vi "HasNext.vi"(8 "error in (no error)":errorcluster, 11 "CompositeIterator":refnum<class "CompositeIterator.lvclass">) -> (0 "error out":errorcluster, 2 "HasNext?(False)":bool, 3 "CompositeIterator Out":refnum<class "CompositeIterator.lvclass">)   [LabVIEW 2015, in "CompositeIterator.lvclass"]
uses:
  CompositeIterator.lvclass
  Interface/Iterator.lvclass
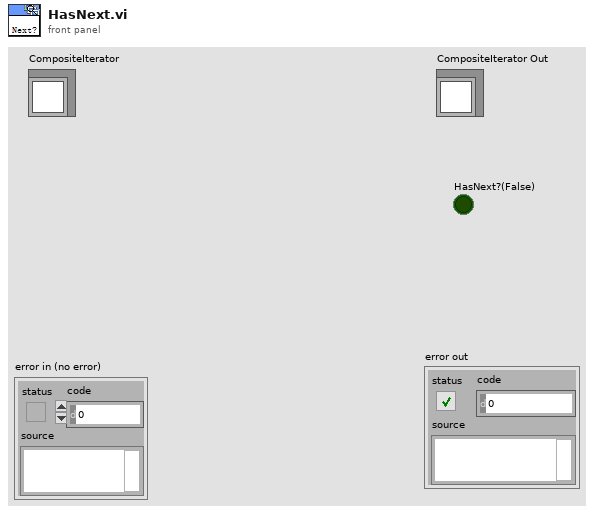
[diagram p1: front panel]
types:
  T1 = typedef "CompositeIterator.lvclass/ObjectAttributes.ctl" = cluster{"Stack":refnum<queue>}
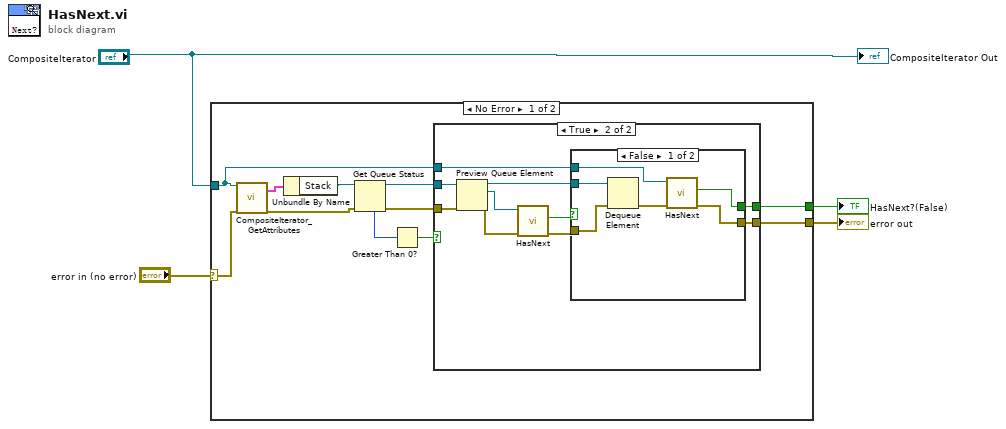
[diagram p0: block diagram]
diagram:
  n1 = case shown="No Error" "error in (no error)" {
    selector: "error in (no error)" -> [w7 w36]
    tunnel: "CompositeIterator" -> [w8 _]
    tunnel: [w11 _] -> w4
    tunnel: [w10 w36] -> w3
    frame No Error {
      n2 = call "CompositeIterator_GetAttributes.vi"("reference in"=w8, "error in (no error)"=w7) -> ("Data"=w6:T1, "error out"=w5:errorcluster)  [unwired: 14 in, 2 out]
      n3 = Unbundle By Name(w6) -> ("Stack"=w9:refnum<queue>)
      n4 = Get Queue Status(queue=w9, error in (no error)=w5) -> (queue out=w12:refnum<queue>, error out=w13:errorcluster, # elements in queue=w15:i32)  [unwired: 1 in, 5 out]
      n5 = Greater Than 0?(x=w15) -> (x > 0?=w14:bool)
      n6 = case shown="True" w14 {
        selector: w14 -> [w17 _]
        tunnel: w13 -> [w16 w26]
        tunnel: w12 -> [_ w27]
        tunnel: [w17 w24] -> w11
        tunnel: [w16 w23] -> w10
        tunnel: w8 -> [_ w22]
        frame False {
        }
        frame True {
          n7 = Preview Queue Element(queue=w27, error in (no error)=w26) -> (queue out=w25:refnum<queue>, element=w21:refnum<class "Iterator.lvclass">, error out=w20:errorcluster)  [unwired: 1 in, 1 out]
          n8 = call-dynamic "HasNext.vi"("error in (no error)"=w20, "Iterator"=w21) -> ("error out"=w18:errorcluster, "HasNext?(False)"=w19:bool)  [unwired: 7 in, 1 out]
          n9 = case shown="False" w19 {
            selector: w19 -> [_ w34]
            tunnel: w18 -> [w33 w35]
            tunnel: w25 -> [w32 _]
            tunnel: [w28 w34] -> w24
            tunnel: [w29 w35] -> w23
            tunnel: w22 -> [w31 _]
            frame False {
              n10 = Dequeue Element(queue=w32, error in (no error)=w33) -> (error out=w30:errorcluster)  [unwired: 1 in, 3 out]
              n11 = call-dynamic "HasNext.vi"("error in (no error)"=w30, "CompositeIterator"=w31) -> ("error out"=w29:errorcluster, "HasNext?(False)"=w28:bool)  [unwired: 7 in, 1 out]
            }
            frame True {
            }
          }
        }
      }
    }
    frame Error {
    }
  }
  "HasNext?(False)" <- w4
  "error out" <- w3
  "CompositeIterator Out" <- "CompositeIterator"
